vi "Actor Core.vi"(8 "error in":errorcluster, 11 "Nested in":refnum<class "GUI Actor.lvclass">) -> (0 "error out":errorcluster, 3 "Actor out":refnum<class "Actor.lvclass">)   [LabVIEW 2019, in "GUI Actor.lvlib" / "GUI Actor.lvclass"]
doc: "(<B>Filename</B>: Actor Framework.lvlib:Actor.lvclass:Actor Core.vi)\n\nReceives messages to the actor, reacts to them, and initiates any error handling that may shut the actor down.\n\nDescendant classes may override this VI to append parallel tasks for the actor to complete while it handles messages. Overrides use the Call Parent Method node."
uses:
  GUI Actor.lvclass
  C:/Program Files (x86)/National Instruments/LabVIEW 2019/vi.lib/ActorFramework/Actor/Actor.lvclass
  <vilib>/ActorFramework/Actor/Actor.lvclass
  Measurment Actor/Measurment Actor/Measurment Actor.lvclass
  Logging/Logging/Logging.lvclass
  GUI Actor.lvclass/GUI Actor.ctl
  <vilib>/ActorFramework/Actor/Actor.lvclass/Actor.ctl
  <vilib>/ActorFramework/Message Enqueuer/Message Enqueuer.lvclass/Message Enqueuer.ctl
  GUI Actor Messages/StartStopACQ Msg/StartStopACQ Msg.lvclass/StartStopACQ Msg.ctl
  GUI Actor Messages/LogEnable Msg/LogEnable Msg.lvclass/LogEnable Msg.ctl
  GUI Actor Messages/File Path Msg/File Path Msg.lvclass/File Path Msg.ctl
  Measurment Actor/Measurment Actor Messages/Amplitud Msg/Amplitud Msg.lvclass/Amplitud Msg.ctl
  Measurment Actor/Measurment Actor Messages/Frecuencia Msg/Frecuencia Msg.lvclass/Frecuencia Msg.ctl
  <vilib>/ActorFramework/Message Enqueuer/Init from Existing Queue.vi
  <vilib>/ActorFramework/Message Enqueuer/Enqueue.vi
  <vilib>/ActorFramework/Stop Msg/Stop Msg.lvclass
  C:/Program Files (x86)/National Instruments/LabVIEW 2019/vi.lib/ActorFramework/Message/Message.lvclass
  GUI Actor Messages/StartStopACQ Msg/StartStopACQ Msg.lvclass
  GUI Actor Messages/LogEnable Msg/LogEnable Msg.lvclass
  GUI Actor Messages/File Path Msg/File Path Msg.lvclass
  Measurment Actor/Measurment Actor Messages/Amplitud Msg/Amplitud Msg.lvclass
  Measurment Actor/Measurment Actor Messages/Frecuencia Msg/Frecuencia Msg.lvclass
  <vilib>/ActorFramework/Message Priority Queue/Priority Enqueue.vi
  <vilib>/ActorFramework/Message Enqueuer/Message Enqueuer.lvclass
  GUI Actor Messages/SelectFormatFile Msg/SelectFormatFile Msg.lvclass
panel:
  out "Waveform Chart":waveform(dbl)(graph)
  in  "Frecuencia":dbl
  in  "Tipo de señal":u16(ring) items=["Cuadrada", "Senoidal", "Triangular"]
  in  "Amplitud":dbl
  in  "Forma":enum16{"txt", "CSV"}(ring)
  in  "Path":path
  in  "Save":bool
  in  "Stop":bool
  in  "Start":bool
  in  "Exit":bool
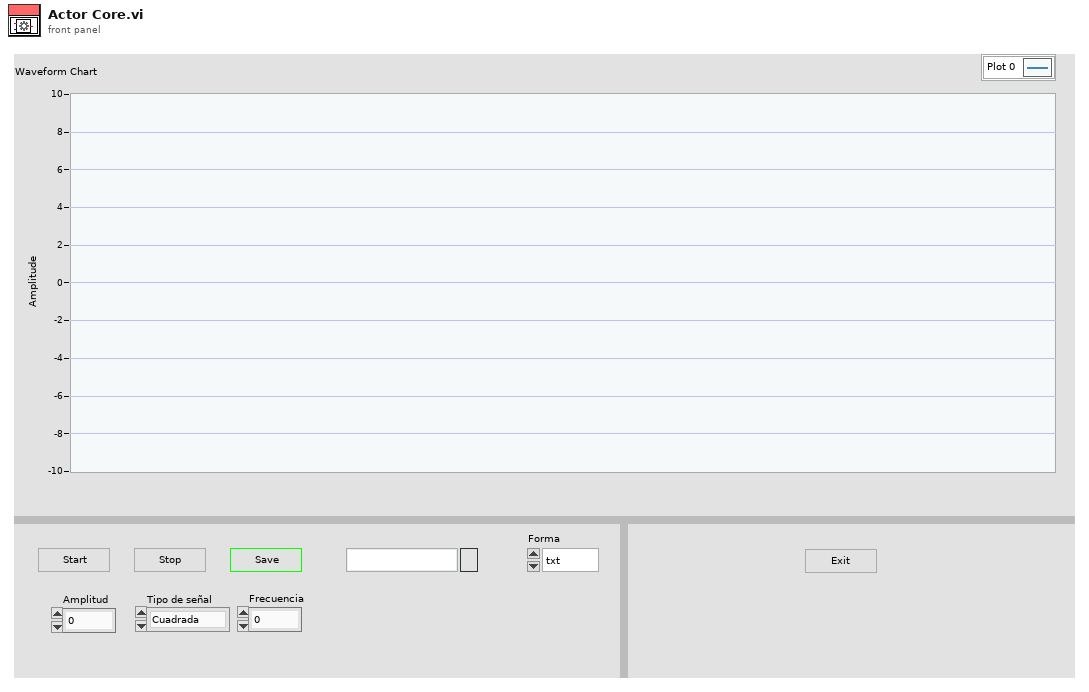
[diagram p1: front panel]
types:
  T1 = cluster{"Stop":refnum<user-event>, "Waveform Chart":refnum<user-event>}
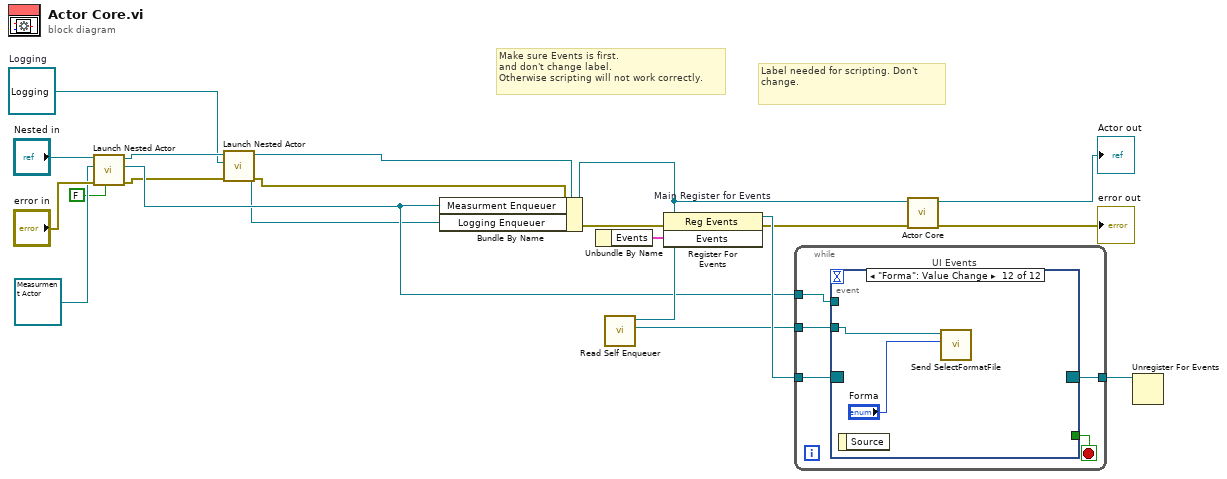
[diagram p0: block diagram]
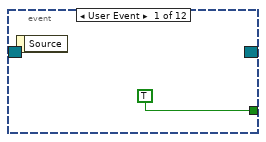
[diagram p2: hidden frame]
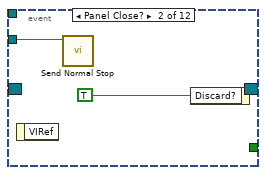
[diagram p3: hidden frame]
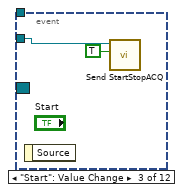
[diagram p4: hidden frame]
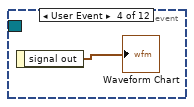
[diagram p5: hidden frame]
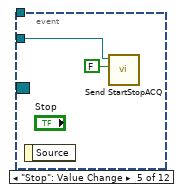
[diagram p6: hidden frame]
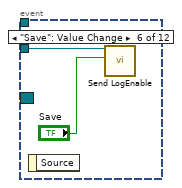
[diagram p7: hidden frame]
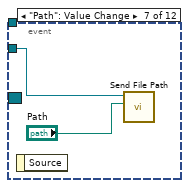
[diagram p8: hidden frame]
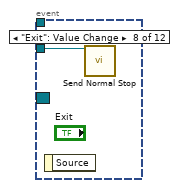
[diagram p9: hidden frame]
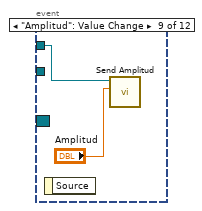
[diagram p10: hidden frame]
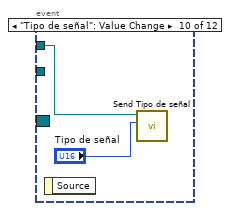
[diagram p11: hidden frame]
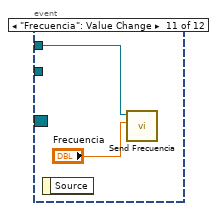
[diagram p12: hidden frame]
diagram:
  w2 = refnum<class "Logging.lvclass"> refnum  # Logging
  # "Label needed for scripting. Don't change."
  # "Make sure Events is first.\nand don't change label.\nOtherwise scripting will not work correctly."
  n1 = call <vilib>:"Launch Nested Actor.vi"("Open Actor Core front panel? (F)"=FALSE, "error in (no error)"="error in", "Nested Actor"=refnum<class "Measurment Actor.lvclass"> refnum ("Measurment Actor.lvlib:Measurment Actor.lvclass"), "Caller Actor in"="Nested in") -> ("error out"=w4:errorcluster, "Nested Actor's Enqueuer"=w7:refnum<class "Message Enqueuer.lvclass">, "Caller Actor out"=w6:refnum<class "GUI Actor.lvclass">)  [unwired: 5 in]
  n2 = call <vilib>:"Launch Nested Actor.vi"("error in (no error)"=w4, "Nested Actor"=w2, "Caller Actor in"=w6) -> ("error out"=w3:errorcluster, "Nested Actor's Enqueuer"=w1:refnum<class "Message Enqueuer.lvclass">, "Caller Actor out"=w5:refnum<class "GUI Actor.lvclass">)  [unwired: 6 in]
  n3 = Bundle By Name(cluster=w5, "Measurment Enqueuer"=w7, "Logging Enqueuer"=w1) -> (w8:refnum<class "GUI Actor.lvclass">)
  n4 = Unbundle By Name(w8) -> ("Events"=w16:T1)
  n5 = call <vilib>:"Read Self Enqueuer.vi"("Actor"=w8) -> ("Self Enqueuer"=w14:refnum<class "Message Enqueuer.lvclass">)  [unwired: 10 in]
  n6 = register-events "Main Register for Events"(error in=w3, w16) -> (reference out=w17:refnum<event-registration>, error out=w13:errorcluster)  [unwired: 1 in]
  n7 = while {
    tunnel: w17 -> [w24]
    tunnel: [w22] -> w15
    tunnel: w14 -> [w21]
    tunnel: w7 -> [w20]
    stop <- w23 stop-if-true
    n8 = event "UI Events" shown="[11] \"Forma\": Value Change" {
      selector: w24 -> [_ _ _ _ _ _ _ _ _ _ _ _]
      dyn-events: [_ _ _ _ _ _ _ _ _ _ _ _] -> w22
      timeout: _ -> [_ _ _ _ _ _ _ _ _ _ _ _]
      tunnel: [TRUE _ _ _ _ _ _ _ _ _ _ _] -> w23
      tunnel: w21 -> [_ w26 w29 _ w31 w33 w35 w37 _ _ _ w45]
      tunnel: w20 -> [_ _ _ _ _ _ _ _ w38 w41 w43 _]
      event User Event {
        n9 = event-data() -> ()  [unwired: 1 in, 1 out]
      }
      event Panel Close? {
        n10 = event-data() -> ()  [unwired: 1 in, 1 out]
        n11 = call <vilib>:"Send Normal Stop.vi"("Message Enqueuer"=w26) -> ()  [unwired: 10 in, 1 out]
        n12 = event-data("Discard?"=TRUE) -> ()  [unwired: 1 in, 1 out]
      }
      event "Start": Value Change {
        n13 = event-data() -> ()  [unwired: 1 in, 1 out]
        n14 = call "Send StartStopACQ.vi"("Start Stop"=TRUE, "Message Enqueuer"=w29) -> ()  [unwired: 8 in, 2 out]
      }
      event User Event {
        n15 = event-data() -> ("signal out"=→"Waveform Chart":waveform(dbl))  [unwired: 1 in]
      }
      event "Stop": Value Change {
        n16 = event-data() -> ()  [unwired: 1 in, 1 out]
        n17 = call "Send StartStopACQ.vi"("Start Stop"=FALSE, "Message Enqueuer"=w31) -> ()  [unwired: 8 in, 2 out]
      }
      event "Save": Value Change {
        n18 = event-data() -> ()  [unwired: 1 in, 1 out]
        n19 = call "Send LogEnable.vi"("Log?"="Save", "Message Enqueuer"=w33) -> ()  [unwired: 8 in, 2 out]
      }
      event "Path": Value Change {
        n20 = event-data() -> ()  [unwired: 1 in, 1 out]
        n21 = call "Send File Path.vi"("Path"="Path", "Message Enqueuer"=w35) -> ()  [unwired: 8 in, 2 out]
      }
      event "Exit": Value Change {
        n22 = event-data() -> ()  [unwired: 1 in, 1 out]
        n23 = call <vilib>:"Send Normal Stop.vi"("Message Enqueuer"=w37) -> ()  [unwired: 10 in, 1 out]
      }
      event "Amplitud": Value Change {
        n24 = event-data() -> ()  [unwired: 1 in, 1 out]
        n25 = call "Send Amplitud.vi"("Amplitud"="Amplitud", "Message Enqueuer"=w38) -> ()  [unwired: 8 in, 2 out]
      }
      event "Tipo de señal": Value Change {
        n26 = event-data() -> ()  [unwired: 1 in, 1 out]
        n27 = call "Send Tipo de señal.vi"("Tipo de señal"="Tipo de señal", "Message Enqueuer"=w41) -> ()  [unwired: 8 in, 2 out]
      }
      event "Frecuencia": Value Change {
        n28 = event-data() -> ()  [unwired: 1 in, 1 out]
        n29 = call "Send Frecuencia.vi"("Frecuencia"="Frecuencia", "Message Enqueuer"=w43) -> ()  [unwired: 8 in, 2 out]
      }
      event "Forma": Value Change {
        n30 = event-data() -> ()  [unwired: 1 in, 1 out]
        n31 = call "Send SelectFormatFile.vi"("Forma"="Forma", "Message Enqueuer"=w45) -> ()  [unwired: 8 in, 2 out]
      }
    }
  }
  n32 = call-parent "Actor Core.vi"("error in"=w13, "Actor in"=w8) -> ("error out"=→"error out":errorcluster, "Actor out"=→"Actor out":refnum<class "Actor.lvclass">)  [unwired: 8 in]
  n33 = Unregister For Events(event registration refnum=w15) -> ()  [unwired: 1 in, 1 out]
